vi "Periodic Tasks.vi"(8 "error in":errorcluster) -> ()   [LabVIEW 2013]
doc: "This VI runs in parallel to other tasks. It can contain as many user-defined periodic loops as you need. These can carry out PID or other sorts of timed response."
uses:
  <vilib>/Rock Robotics/SystemInterfaces/Utilities/FPGA_UtilitiesLED Source.ctl
  <vilib>/Rock Robotics/SystemInterfaces/Utilities/FPGA_UtilitiesLED State.ctl
  <vilib>/Rock Robotics/WPI/Relay/WPI_RelayValue.ctl
  <vilib>/Rock Robotics/WPI/Joystick/WPI_JoystickGetSetRefNum.vi
  Robot Global Data.vi
  <vilib>/Rock Robotics/WPI/RobotDrive/WPI_RobotDriveGetSetRefNum.vi
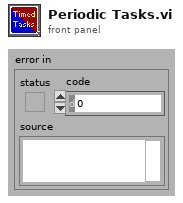
[diagram p1: front panel]
types:
  T1 = typedef "WPI_CompressorDevRef.ctl" = cluster{"DevStatus":errorcluster, "DigitalInputDevRef":T2, "RelayDevRef":T5}
  T2 = typedef "WPI_DigitalInputDevRef.ctl" = cluster{"DevStatus":errorcluster, "DIO Channel":T3, "Digital Module":T4}
  T3 = typedef "FPGA_DIOChannel.ctl" = enum8{"DIO 1", "DIO 2", "DIO 3", "DIO 4", "DIO 5", "DIO 6", "DIO 7", "DIO 8", "DIO 9", "DIO 10", "DIO 11", "DIO 12", "DIO 13", "DIO 14", "Invalid"}
  T4 = typedef "FPGA_TypedefDigitalModule.ctl" = enum16{"Digital Module 1", "Digital Module 2"}
  T5 = typedef "WPI_RelayDevRef.ctl" = cluster{"DevStatus":errorcluster, "Relay Channel":T6, "Digital Module":T4, "Relay Direction":T7}
  T6 = typedef "FPGA_DIORelayChannel.ctl" = enum8{"Relay 1", "Relay 2", "Relay 3", "Relay 4", "Relay 5", "Relay 6", "Relay 7", "Relay 8", "Invalid"}
  T7 = typedef "WPI_RelayDirection.ctl" = enum16{"Both directions", "Forward only", "Reverse only"}
  T8 = typedef "FPGA_UtilitiesLED State.ctl" = enum16{"Off", "On", "Toggle"}
  T9 = typedef "FPGA_UtilitiesLED Source.ctl" = enum16{"User LED", "FPGA LED"}
  T10 = cluster{"Position":cluster{"X":dbl, "Y":dbl}, "Distance (ft)":dbl}[]
  T11 = typedef "WPI_EncoderDevRef.ctl" = cluster{"DevStatus":errorcluster, "EncoderIndex":T12, "CounterIndex":T13, "DistancePerCount":dbl, "Decoding Type":T14}
  T12 = typedef "FPGA_EncoderIdx.ctl" = enum8{"Enc 0", "Enc 1", "Enc 2", "Enc 3", "Invalid"}
  T13 = typedef "FPGA_CounterCtrSystemIndex.ctl" = enum8{"Ctr 0", "Ctr 1", "Ctr 2", "Ctr 3", "Ctr 4", "Ctr 5", "Ctr 6", "Ctr 7", "Invalid"}
  T14 = typedef "WPI_EncoderType.ctl" = enum16{"1x", "2x", "4x"}
  T15 = typedef "WPI_RobotDriveDevRef.ctl" = cluster{"DevStatus":errorcluster, "Motors[]":T16[], "Square Inputs":bool, "Max Output":dbl, "Isochronous":bool}
  T16 = typedef "WPI_MotorControlDeviceRef.ctl" = cluster{"DeviceStatus":errorcluster, "Type":enum16{"PWM", "CAN"}, "PWM":cluster{"Digital Module":T4, "PWM Channel":T17, "DeadBand":T18}, "CAN":cluster{"Device Number":u8, "Control Mode":T19, "Semaphore":T20, "Max Vout":dbl}, "Invert":bool, "TransformRef":T21, "InvTransformRef":T21}
  T17 = typedef "FPGA_DIOPWMChannel.ctl" = enum8{"PWM 1", "PWM 2", "PWM 3", "PWM 4", "PWM 5", "PWM 6", "PWM 7", "PWM 8", "PWM 9", "PWM 10", "Invalid"}
  T18 = typedef "WPI_PWMDeadband.ctl" = cluster{"Name":string, "maxPositivePwm":i32, "minPositivePwm":i32, "centerPwm":i32, "maxNegativePwm":i32, "minNegativePwm":i32, "angularRange":u16}
  T19 = typedef "WPI_CANJaguar_ControlMode.ctl" = enum8{"Percent VBus", "Current", "Speed", "Position", "Voltage"}
  T20 = typedef "Semaphore RefNum" = refnum<k1>
  T21 = typedef "WPI_PWMTransform_ConPane.ctl" = refnum<vi>
  T22 = typedef "WPI_JoystickDevRef.ctl" = cluster{"Device":T23}
  T23 = typedef "WPI_JoystickDeviceEnum.ctl" = enum16{"USB 1", "USB 2", "USB 3", "USB 4", "Kinect 1", "Kinect 2"}
  T24 = cluster{"JoystickDevRef":T22, "RobotDriveDevRef":T15}
  T25 = typedef "WPI_GyroDevRef.ctl" = cluster{"DevStatus":errorcluster, "Analog Module":T26, "Analog Channel":T27, "Offset":dbl, "Gain (VoltsPerDegree/Second)":dbl}
  T26 = typedef "FPGA_TypedefAnalogModule.ctl" = enum16{"Analog Module 1", "Analog Module 2"}
  T27 = typedef "FPGA_AIChannel.ctl" = enum8{"AI 1", "AI 2", "AI 3", "AI 4", "AI 5", "AI 6", "AI 7", "AI 8", "Invalid"}
  T28 = typedef "WPI_RelayValue.ctl" = enum16{"Off", "On", "Forward", "Reverse"}
  T29 = cluster{"axis 1 (x)":dbl, "axis 2 (y)":dbl, "axis 3 (throttle)":dbl, "axis 4":dbl, "axis 5":dbl, "axis 6":dbl}
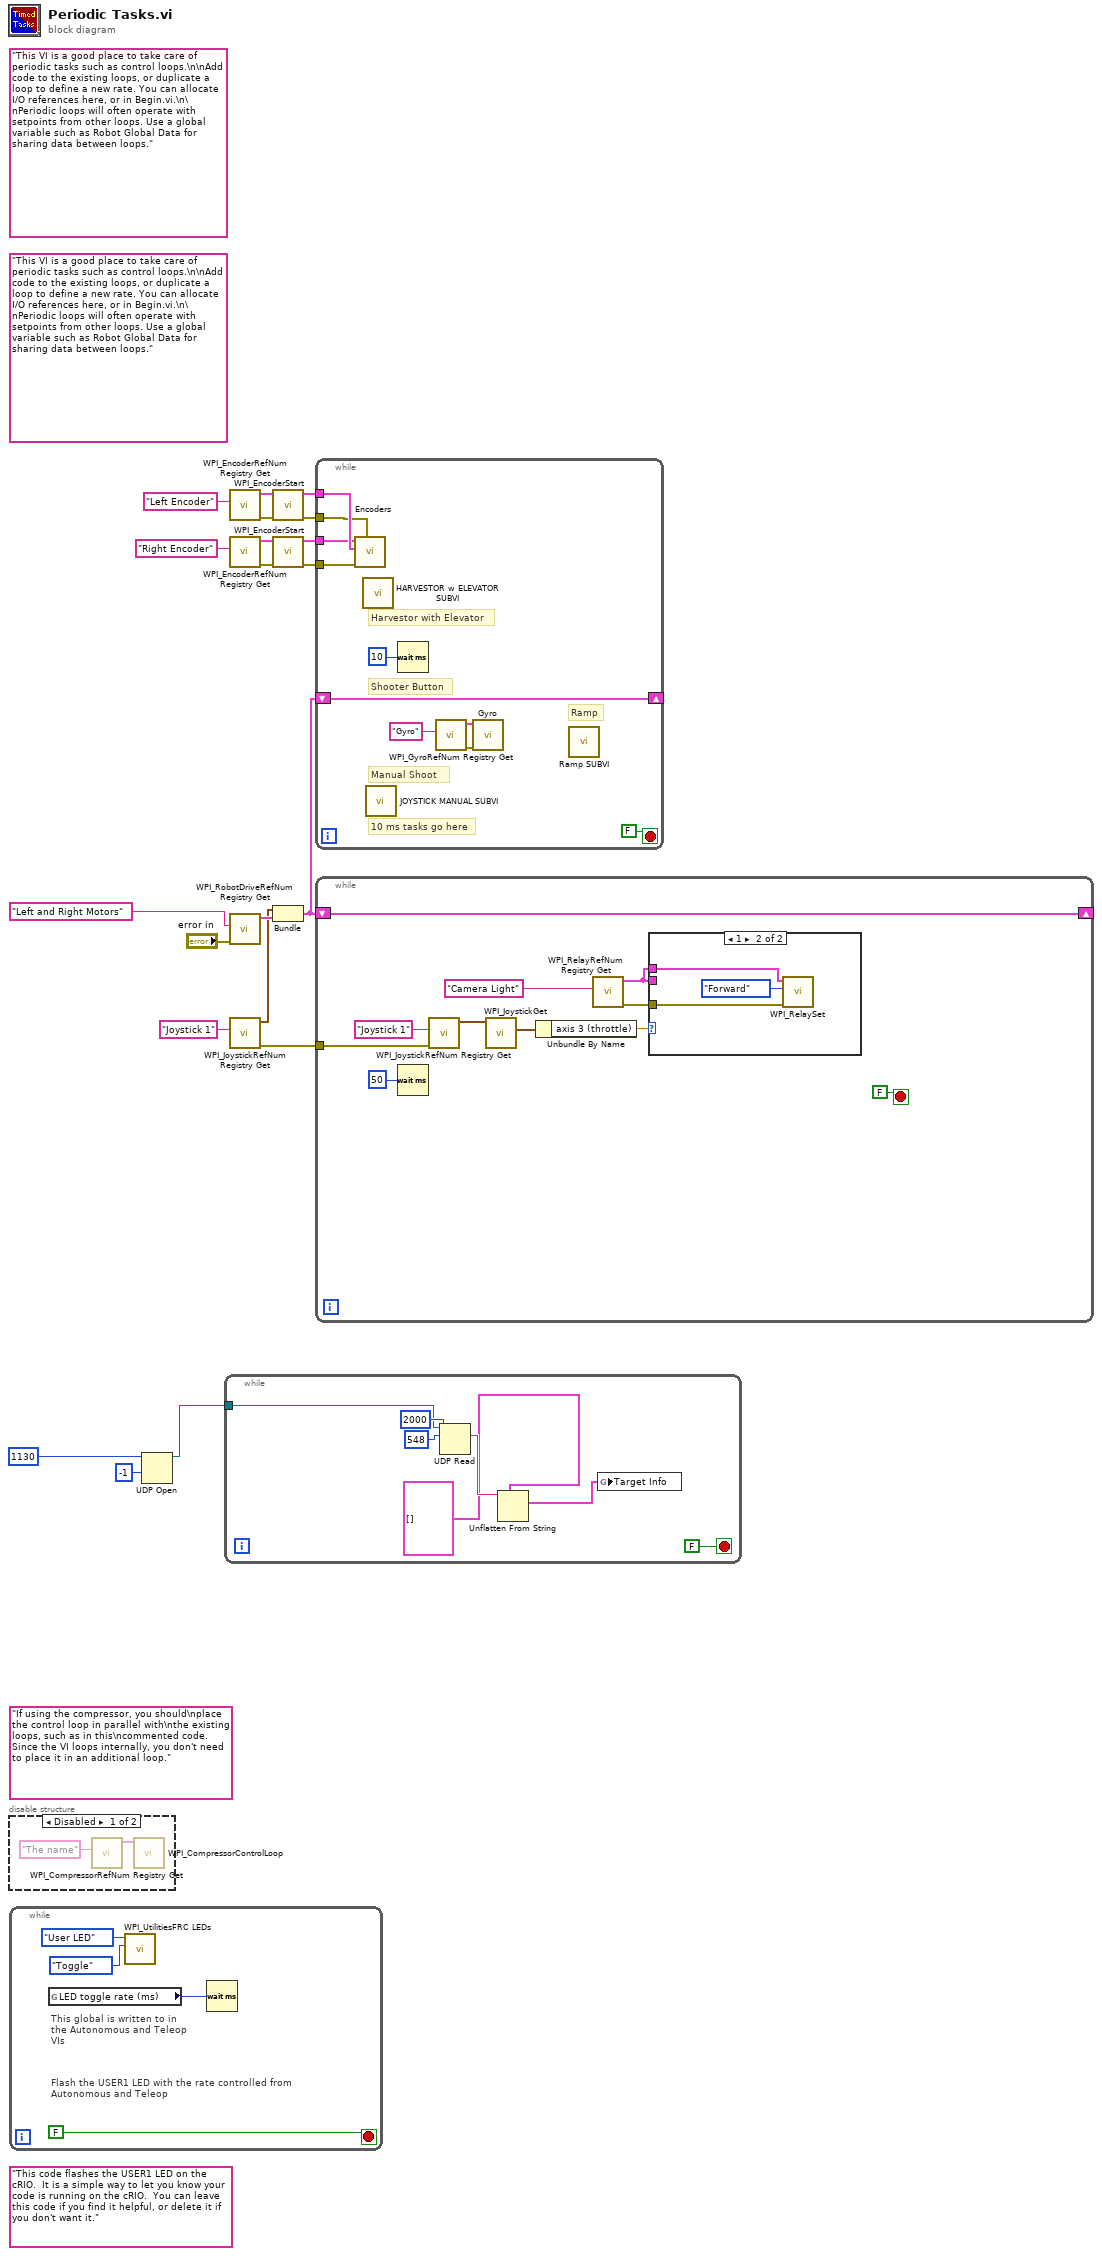
[diagram p0: block diagram]
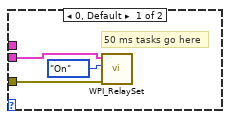
[diagram p3: hidden frame]
diagram:
  (unwired) "This VI is a good place to take care of periodic tasks such as control loops.\n\nAdd code to the existing loops, or duplicate a loop to define a new rate. You can allocate I/O references here, or in Begin.vi.\n\nPeriodic loops will often operate with setpoints from other loops. Use a global variable such as Robot Global Data for sharing data between loops."
  (unwired) "If using the compressor, you should\nplace the control loop in parallel with\nthe existing loops, such as in this\ncommented code. Since the VI loops internally, you don't need to place it in an additional loop."
  (unwired) "This code flashes the USER1 LED on the cRIO.  It is a simple way to let you know your code is running on the cRIO.  You can leave this code if you find it helpful, or delete it if you don't want it."
  (unwired) "This VI is a good place to take care of periodic tasks such as control loops.\n\nAdd code to the existing loops, or duplicate a loop to define a new rate. You can allocate I/O references here, or in Begin.vi.\n\nPeriodic loops will often operate with setpoints from other loops. Use a global variable such as Robot Global Data for sharing data between loops."
  n1 = disable-structure shown="Disabled" {
    frame Disabled {
      n2 = call <vilib>:"WPI_CompressorRefNum Registry Get.vi"("refnum name"="The name") -> ("CompressorDevRef"=w22:T1)  [unwired: 9 in, 1 out]
      n3 = call <vilib>:"WPI_CompressorControlLoop.vi"("CompressorDevRef"=w22) -> ()  [unwired: 11 in]
    }
    frame Enabled {
    }
  }
  n4 = while {
    stop <- FALSE stop-if-true
    # "This global is written to in the Autonomous and Teleop VIs"
    # "Flash the USER1 LED with the rate controlled from Autonomous and Teleop"
    n5 = global read "Robot Global Data.vi" "LED toggle rate (ms)"() -> (w23:u32)
    n6 = call <vilib>:"WPI_UtilitiesFRC LEDs.vi"("State"=FPGA_UtilitiesLED_State."Toggle", "LED Type"=FPGA_UtilitiesLED_Source."User LED") -> ()  [unwired: 1 in, 9 out]
    n7 = Wait (ms)(milliseconds to wait=w23) -> ()  [unwired: 1 out]
  }
  n8 = UDP Open(9:-1 ("timeout ms (25000)"), 11:u16 1130 ("port")) -> (port=w1:refnum<k16>)  [unwired: 3 in, 2 out]
  n9 = while {
    tunnel: w1 -> [w30]
    stop <- FALSE stop-if-true
    n10 = UDP Read(connection ID=w30, max size (548)=548, timeout ms (25000)=2000) -> (data out=w31:string)  [unwired: 1 in, 4 out]
    n11 = Unflatten From String(type=T10 [] ("Target Info"), binary string=w31) -> (value=w27:T10)  [unwired: 3 in, 2 out]
    n12 = global write "Robot Global Data.vi" "Target Info"(w27) -> ()
  }
  n13 = call <vilib>:"WPI_EncoderRefNum Registry Get.vi"("refnum name"="Left Encoder") -> ("error out"=w9:errorcluster, "EncoderDevRef"=w10:T11)  [unwired: 1 in, 8 out]
  n14 = call <vilib>:"WPI_EncoderRefNum Registry Get.vi"("refnum name"="Right Encoder") -> ("error out"=w12:errorcluster, "EncoderDevRef"=w11:T11)  [unwired: 1 in, 8 out]
  n15 = call <vilib>:"WPI_RobotDriveRefNum Registry Get.vi"("error in (no error)"="error in", "refnum name"="Left and Right Motors") -> ("RobotDriveDevRef"=w18:T15)  [unwired: 9 out]
  n16 = call <vilib>:"WPI_JoystickRefNum Registry Get.vi"("refnum name"="Joystick 1") -> ("error out"=w4:errorcluster, "JoystickDevRef"=w15:T22)  [unwired: 1 in, 8 out]
  n17 = call <vilib>:"WPI_EncoderStart.vi"("error in (no error)"=w9, "EncoderDevRef"=w10) -> ("error out"=w5:errorcluster, "EncoderDevRef"=w8:T11)  [unwired: 8 out]
  n18 = call <vilib>:"WPI_EncoderStart.vi"("error in (no error)"=w12, "EncoderDevRef"=w11) -> ("error out"=w6:errorcluster, "EncoderDevRef"=w7:T11)  [unwired: 8 out]
  n19 = Bundle("JoystickDevRef"=w15, "RobotDriveDevRef"=w18) -> (w17:T24)  [unwired: 1 out]
  n20 = while {
    shift-right: [w41] -> _
    shift-left: w17 -> [w41]
    tunnel: w8 -> [w37]
    tunnel: w7 -> [w36]
    tunnel: w6 -> [w35]
    tunnel: w5 -> [w34]
    stop <- FALSE stop-if-true
    # "Manual Shoot"
    # "Harvestor with Elevator"
    # "Shooter Button"
    # "Ramp"
    # "10 ms tasks go here"
    n21 = call "Encoders.vi"("error in (no error) 2"=w34, "error in (no error)"=w35, "Left Encoder"=w37, "Right Encoder"=w36) -> ()  [unwired: 8 out]
    n22 = call "HARVESTOR w ELEVATOR  SUBVI.vi"() -> ()  [unwired: 12 in]
    n23 = call "JOYSTICK MANUAL SUBVI.vi"() -> ()  [unwired: 12 in]
    n24 = Wait (ms)(milliseconds to wait=u32 10) -> ()  [unwired: 1 out]
    n25 = call <vilib>:"WPI_GyroRefNum Registry Get.vi"("refnum name"="Gyro") -> ("error out"=w39:errorcluster, "GyroDevRef"=w38:T25)  [unwired: 1 in, 8 out]
    n26 = call "Gyro.vi"("error in (no error)"=w39, "GyroDevRef"=w38) -> ()  [unwired: 10 out]
    n27 = call "Ramp SUBVI.vi"() -> ()  [unwired: 12 in]
  }
  n28 = while {
    shift-right: [w53] -> _
    shift-left: w17 -> [w53]
    tunnel: w4 -> [w44]
    stop <- FALSE stop-if-true
    n29 = Wait (ms)(milliseconds to wait=u32 50) -> ()  [unwired: 1 out]
    n30 = call <vilib>:"WPI_JoystickRefNum Registry Get.vi"("error in (no error)"=w44, "refnum name"="Joystick 1") -> ("JoystickDevRef"=w47:T22)  [unwired: 8 in, 1 out]
    n31 = call <vilib>:"WPI_JoystickGet.vi"("JoystickDevRef"=w47) -> ("Axes"=w50:T29)  [unwired: 4 in, 2 out]
    n32 = Unbundle By Name(w50) -> ("axis 3 (throttle)"=w51:dbl)
    n33 = call <vilib>:"WPI_RelayRefNum Registry Get.vi"("refnum name"="Camera Light") -> ("error out"=w46:errorcluster, "RelayDevRef"=w45:T5)  [unwired: 9 in]
    n34 = case shown="1" w51 {
      tunnel: w46 -> [w56 w58]
      tunnel: w45 -> [w55 _]
      tunnel: w45 -> [_ w59]
      frame 0, Default {
        # "50 ms tasks go here"
        n35 = call <vilib>:"WPI_RelaySet.vi"("error in (no error)"=w56, "RelayValue"=WPI_RelayValue."On", "RelayDevRef"=w55) -> ()  [unwired: 7 in, 2 out]
      }
      frame 1 {
        n36 = call <vilib>:"WPI_RelaySet.vi"("error in (no error)"=w58, "RelayValue"=WPI_RelayValue."Forward", "RelayDevRef"=w59) -> ()  [unwired: 7 in, 2 out]
      }
    }
  }
